vi "place cursors at crossovers.vi"(7 "index of first cursor":i32, 8 "error in (no error)":errorcluster, 10 "crossovers":dbl[](array[numeric]), 11 "XYGraph in":refnum<vi>) -> (0 "error out":errorcluster)   [LabVIEW 2014]
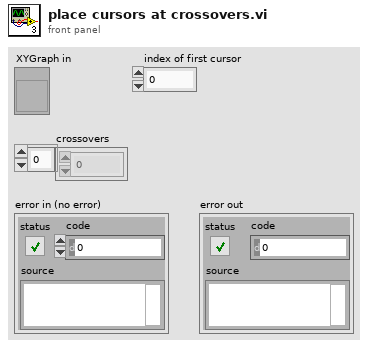
[diagram p1: front panel]
types:
  T1 = typedef "LVCursorListTypeDef.ctl" = cluster{"Name":string, "Color":u32, "Style":u8, "Point Style":u8, "Name Visible":bool, "Allow Drag":bool, "Cursor Mode":u32, "Plot":i32, "Index":i32, "Position":cluster{"X":dbl, "Y":dbl}, "X Scale":u32, "Y Scale":u32, "Watch Plots":i32[], "Watch All Plots":bool, "Plot Area":i32, "Label Offset":cluster{"X":dbl, "Y":dbl}}[]
  T2 = cluster{"Name":string, "Color":u32, "Style":u8, "Point Style":u8, "Name Visible":bool, "Allow Drag":bool, "Cursor Mode":u32, "Plot":i32, "Index":i32, "Position":cluster{"X":dbl, "Y":dbl}, "X Scale":u32, "Y Scale":u32, "Watch Plots":i32[], "Watch All Plots":bool, "Plot Area":i32, "Label Offset":cluster{"X":dbl, "Y":dbl}}
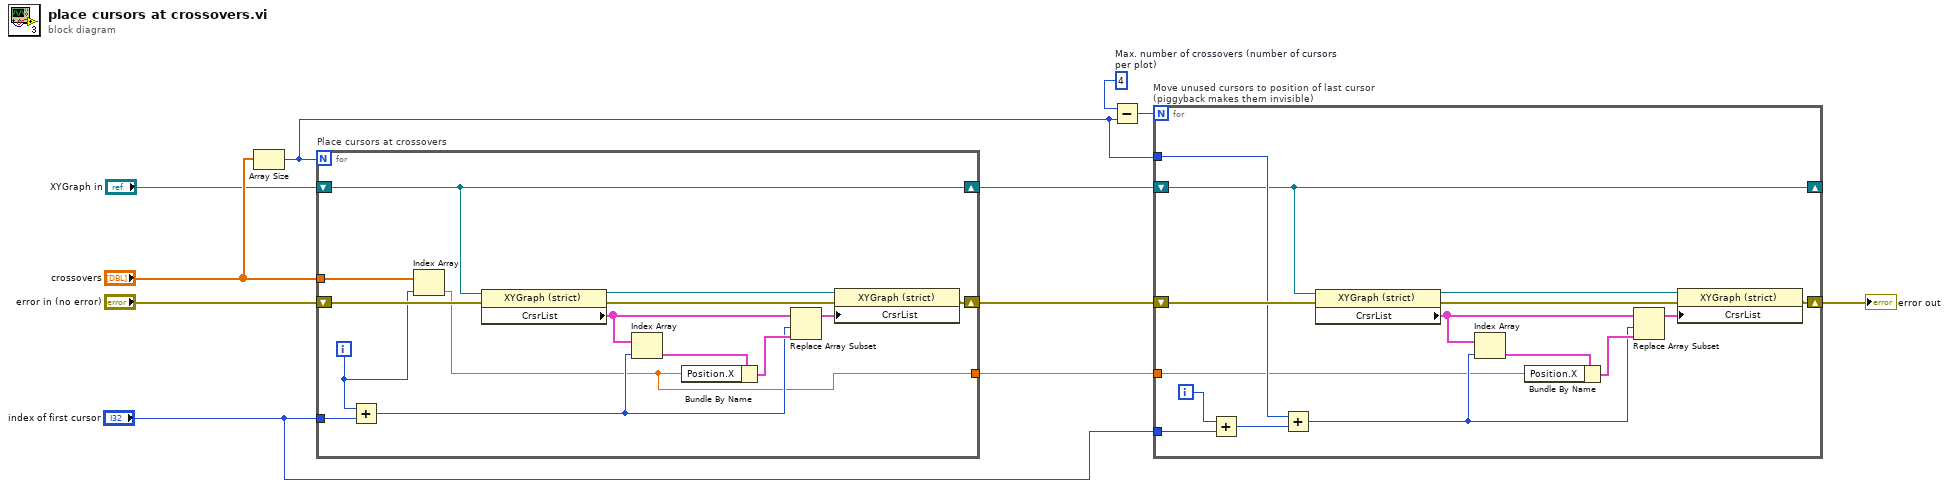
[diagram p0: block diagram]
diagram:
  w8 = 4  # Max. number of crossovers (number of cursors per plot)
  n1 = Array Size(array="crossovers") -> (size(s)=w5:i32)
  n2 = for "Place cursors at crossovers" {
    N: w5 -> [_]
    shift-right: [w20] -> w6
    shift-left: "error in (no error)" -> [w17]
    tunnel: "crossovers" -> [w18]
    shift-right: [w16] -> w4
    shift-left: "XYGraph in" -> [w16]
    tunnel: "index of first cursor" -> [w15]
    tunnel: [w12] -> w1
    i -> [w13]
    n3 = Add(x=w13, y=w15) -> (x+y=w14:i32)
    n4 = Index Array(array=w18, index=w13) -> (element=w12:dbl)
    n5 = property class="XYGraph (strict)"(reference=w16, error in=w17) -> (reference out=w25:refnum<vi>, error out=w19:errorcluster, "CrsrList"=w24:T1)
    n6 = Index Array(array=w24, index=w14) -> (element=w22:T2)
    n7 = Bundle By Name(cluster=w22, "Position.X"=w12) -> (w21:T2)
    n8 = Replace Array Subset(array=w24, new element=w21, index=w14) -> (w23:T1)
    n9 = property class="XYGraph (strict)"(reference=w25, error in=w19, "CrsrList"=w23) -> (error out=w20:errorcluster)  [unwired: 1 out]
  }
  n10 = Subtract(x=w8, y=w5) -> (x-y=w7:i32)
  n11 = for "Move unused cursors to position of last cursor (piggyback makes them invisible)" {
    N: w7 -> [_]
    shift-right: [w35] -> w3
    shift-left: w6 -> [w33]
    tunnel: w5 -> [w32]
    shift-right: [w30] -> _
    shift-left: w4 -> [w30]
    tunnel: "index of first cursor" -> [w29]
    tunnel: w1 -> [w26]
    i -> [w28]
    n12 = Add(x=w28, y=w29) -> (x+y=w27:i32)
    n13 = Add(x=w32, y=w27) -> (x+y=w31:i32)
    n14 = property class="XYGraph (strict)"(reference=w30, error in=w33) -> (reference out=w40:refnum<vi>, error out=w34:errorcluster, "CrsrList"=w39:T1)
    n15 = Index Array(array=w39, index=w31) -> (element=w37:T2)
    n16 = Bundle By Name(cluster=w37, "Position.X"=w26) -> (w36:T2)
    n17 = Replace Array Subset(array=w39, new element=w36, index=w31) -> (w38:T1)
    n18 = property class="XYGraph (strict)"(reference=w40, error in=w34, "CrsrList"=w38) -> (error out=w35:errorcluster)  [unwired: 1 out]
  }
  "error out" <- w3
